vi "1L15_conv_s_en_mns_hrs.vi"(0 "temps en s":i32) -> (1 "Temps en hrs":dbl, 2 "temps en mn":dbl)   [LabVIEW 2010, in "lv_01.lvlib"]
uses:
  lv_01.lvlib
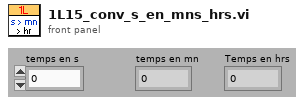
[diagram p1: front panel]
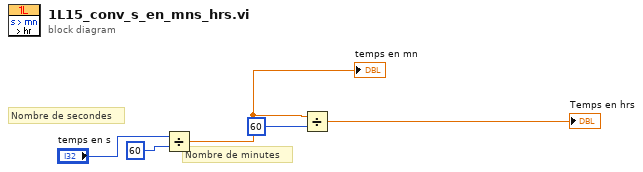
[diagram p0: block diagram]
diagram:
  # "Nombre de minutes"
  # "Nombre de secondes"
  n1 = Divide(x="temps en s", y=60) -> (x/y=w4:dbl)
  "temps en mn" <- w4
  n2 = Divide(x=w4, y=60) -> (x/y=→"Temps en hrs":dbl)
